vi "Calculate_w12.vi"(0 "Data in":fxp<+/-,32,14>[](array[numeric])=[0.0, 0.0, 0.0, 0.0, 0.0, 0.0, 0.0, 0.0], 1 "w12_a":fxp<+/-,32,12>, 2 "w12_b":fxp<+/-,32,14>, 5 "reset":bool, 11 "valid in":bool, 12 "1/dt":fxp<+/-,32,26>=10000000.0 format="%#_45g", 13 "dw scale":i32, 14 "w12 scale":i32) -> (4 "data out":fxp<+/-,32,14>[](array[numeric]), 6 "dw":fxp<+/-,64,48>, 10 "w12":fxp<+/-,64,48>, 15 "valid out":bool)   [LabVIEW 2025]
uses:
  <vilib>/rvi/FXPMathLib/FxpDiv/subVIs/nifxpmath_Div_SimConfig.ctl
  <vilib>/rvi/FXPMathLib/FxpDiv/simVIs/DllFxpDivTemp_sub.vi
  <vilib>/rvi/FXPMathLib/FxpAdd/XNode/nifxpmath_Add.xnode
  <vilib>/rvi/FXPMathLib/FxpSub/XNode/nifxpmath_Sub.xnode
  <vilib>/rvi/FXPMathLib/FxpMul/XNode/nifxpmath_Multiplier.xnode
  <vilib>/rvi/FXPMathLib/FxpReciprocal/XNode/nifxpmath_Reciprocal.xnode
  <vilib>/rvi/FXPMathLib/FxpDiv/XNode/nifxpmath_Div.xnode
  <vilib>/rvi/FXPMathLib/sim/FxpSim.dll
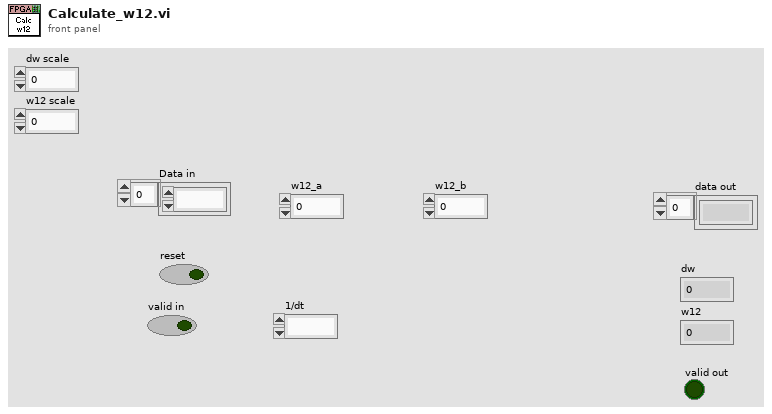
[diagram p1: front panel]
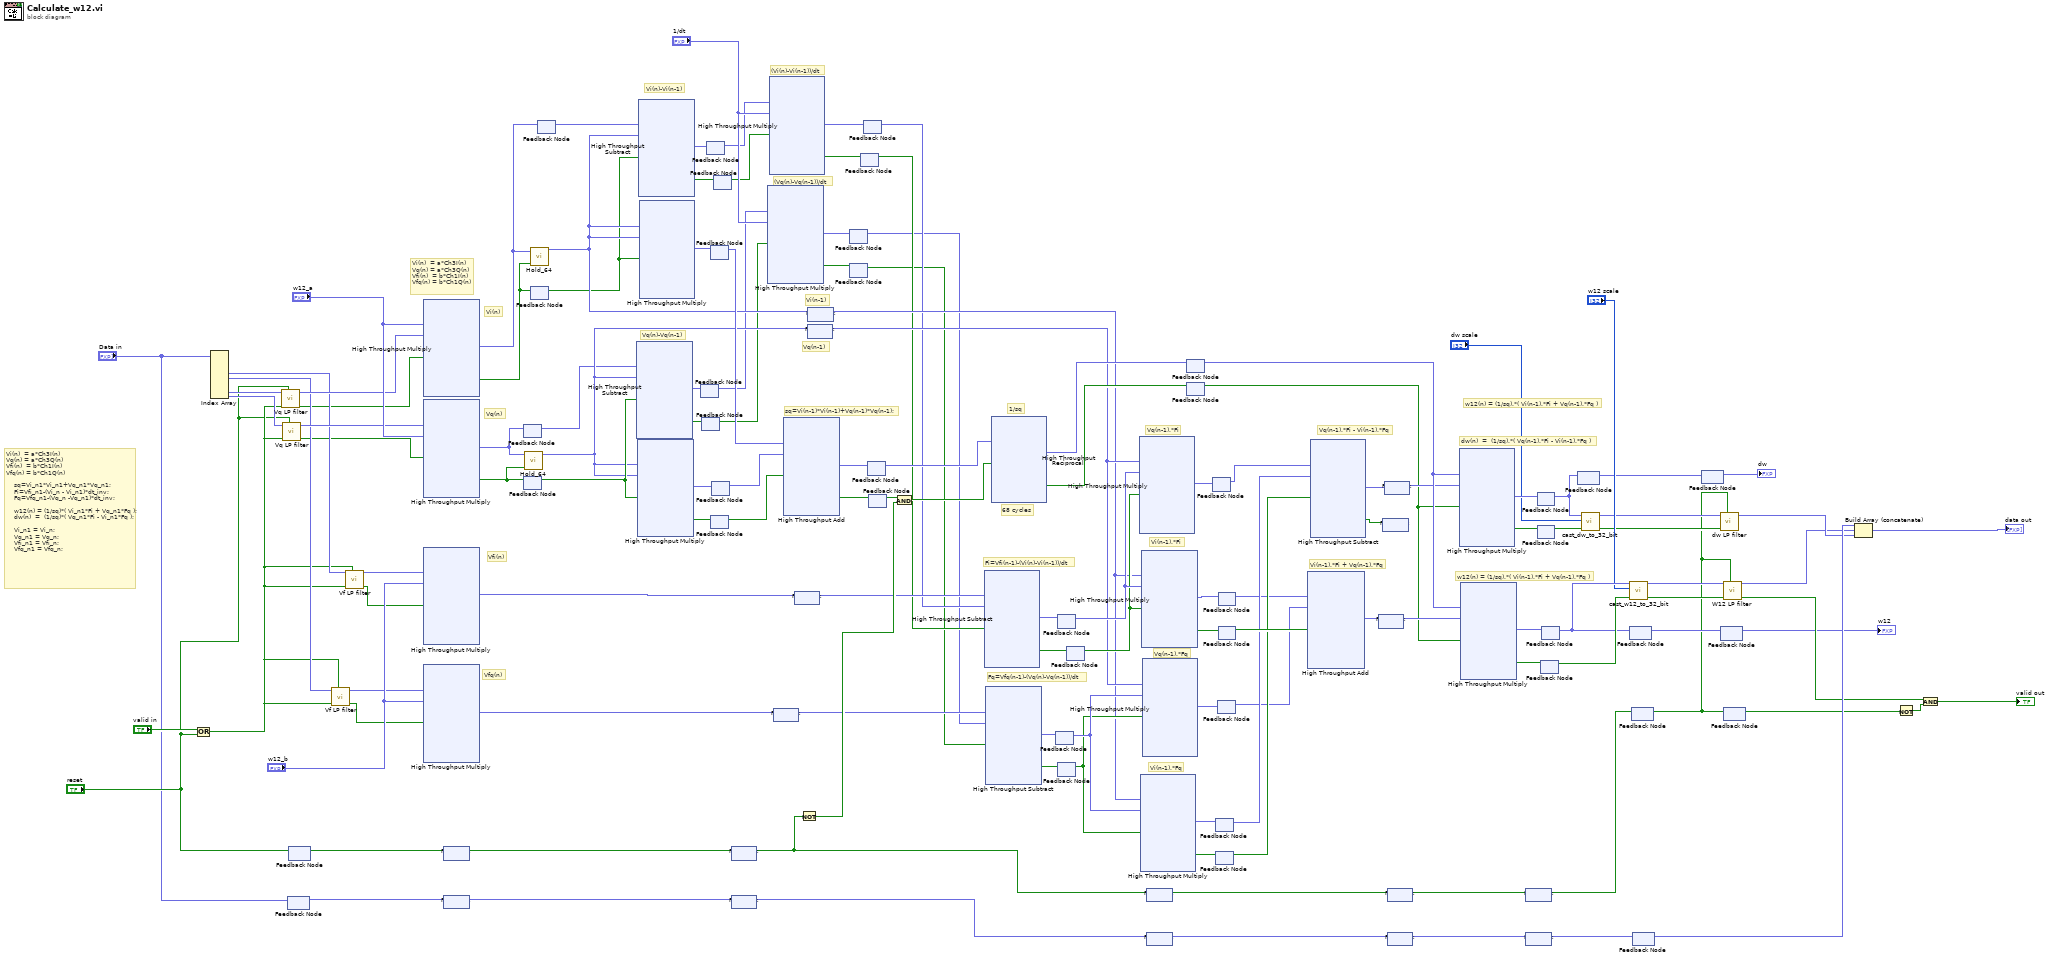
[diagram p0: block diagram]
diagram:
  # "68 cycles"
  # "w12(n) = (1/sq).*( Vi(n-1).*Fi + Vq(n-1).*Fq )"
  # "dw(n)  =  (1/sq).*( Vq(n-1).*Fi - Vi(n-1).*Fq )"
  # "1/sq"
  # "w12(n) = (1/sq).*( Vi(n-1).*Fi + Vq(n-1).*Fq )"
  # "Vq(n-1).*Fi - Vi(n-1).*Fq"
  # "Vi(n-1).*Fi + Vq(n-1).*Fq"
  # "Vi(n-1).*Fq"
  # "Vq(n-1).*Fi"
  # "Vq(n-1).*Fq"
  # "Vq(n-1)"
  # "Vi(n-1)"
  # "Vi(n-1).*Fi"
  # "Fq=Vfq(n-1)-(Vq(n)-Vq(n-1))/dt"
  # "Fi=Vfi(n-1)-(Vi(n)-Vi(n-1))/dt"
  # "(Vq(n)-Vq(n-1))/dt"
  # "(Vi(n)-Vi(n-1))/dt"
  # "Vq(n)-Vq(n-1)"
  # "Vi(n)-Vi(n-1)"
  # "sq=Vi(n-1)*Vi(n-1)+Vq(n-1)*Vq(n-1);"
  # "Vfq(n)"
  # "Vfi(n)"
  # "Vq(n)"
  # "Vi(n)  = a*Ch3I(n)\nVq(n) = a*Ch3Q(n)\nVfi(n)  = b*Ch1I(n)\nVfq(n) = b*Ch1Q(n)"
  # "Vi(n)"
  # "Vi(n)  = a*Ch3I(n)\nVq(n) = a*Ch3Q(n)\nVfi(n)  = b*Ch1I(n)\nVfq(n) = b*Ch1Q(n)\n    \n    sq=Vi_n1*Vi_n1+Vq_n1*Vq_n1;\n    Fi=Vfi_n1-(Vi_n - Vi_n1)*dt_inv;\n    Fq=Vfq_n1-(Vq_n -Vq_n1)*dt_inv;\n    \n    w12(n) = (1/sq)*( Vi_n1*Fi + Vq_n1*Fq );\n    dw(n)  =  (1/sq)*( Vq_n1*Fi - Vi_n1*Fq );\n    \n    Vi_n1 = Vi_n;\n    Vq_n1 = Vq_n;\n    Vfi_n1 = Vfi_n;\n    Vfq_n1 = Vfq_n;"
  n1 = Or(x="valid in", y="reset") -> (x .or. y?=w5:bool)
  n2 = Index Array(array="Data in") -> (element #3=w11:fxp<+/-,32,14>, element #4=w13:fxp<+/-,32,14>, element #7=w17:fxp<+/-,32,14>, element #8=w15:fxp<+/-,32,14>)  [unwired: 8 in, 4 out]
  n3 = call "Vq LP filter.vi"("reset"="reset", "input valid"=w5, "x"=w17) -> ("output valid"=w6:bool, "y"=w16:fxp<+/-,32,14>)  [unwired: 7 in]
  n4 = call "Vq LP filter.vi"("reset"="reset", "input valid"=w5, "x"=w15) -> ("output valid"=w7:bool, "y"=w14:fxp<+/-,32,14>)  [unwired: 7 in]
  n5 = feedback #1() -> (w1:fxp<+/-,32,14>[])  [unwired: 1 in]
  n6 = feedback-in #1("Data in") -> ()
  n7 = feedback #2() -> (w3:bool)  [unwired: 1 in]
  n8 = feedback-in #2("reset") -> ()
  n9 = call "Vf LP filter.vi"("reset"=w5, "input valid"=w5, "x"=w13) -> ("output valid"=w9:bool, "y"=w12:fxp<+/-,32,14>)  [unwired: 7 in]
  n10 = call "Vf LP filter.vi"("reset"=w5, "input valid"=w5, "x"=w11) -> ("output valid"=w8:bool, "y"=w10:fxp<+/-,32,14>)  [unwired: 7 in]
  n11 = xnode ("High Throughput Multiply")("x"="w12_a", "y"=w16, "input valid"=w6) -> ("x*y"=w89:fxp<+/-,64,26>, "output valid"=w88:bool)  [unwired: 1 in, 1 out]
  n12 = xnode ("High Throughput Multiply")("x"=w10, "y"="w12_b", "input valid"=w8) -> ("x*y"=w91:fxp<+/-,64,28>)  [unwired: 1 in, 2 out]
  n13 = xnode ("High Throughput Multiply")("x"=w14, "y"="w12_a", "input valid"=w7) -> ("x*y"=w87:fxp<+/-,64,26>, "output valid"=w86:bool)  [unwired: 1 in, 1 out]
  n14 = xnode ("High Throughput Multiply")("x"=w12, "y"="w12_b", "input valid"=w9) -> ("x*y"=w90:fxp<+/-,64,28>)  [unwired: 1 in, 2 out]
  n15 = feedback #3() -> (w101:bool)  [unwired: 1 in]
  n16 = feedback-in #3(w3) -> ()
  n17 = feedback #4() -> (w100:fxp<+/-,32,14>[])  [unwired: 1 in]
  n18 = feedback-in #4(w1) -> ()
  n19 = feedback #5() -> (w63:fxp<+/-,64,26>)  [unwired: 1 in]
  n20 = feedback-in #5(w87) -> ()
  n21 = feedback #6() -> (w65:bool)  [unwired: 1 in]
  n22 = feedback-in #6(w86) -> ()
  n23 = call "Hold_64.vi"("valid in"=w86, "value in"=w87) -> ("value out"=w64:fxp<+/-,64,26>)  [unwired: 8 in, 1 out]
  n24 = call "Hold_64.vi"("valid in"=w88, "value in"=w89) -> ("value out"=w67:fxp<+/-,64,26>)  [unwired: 8 in, 1 out]
  n25 = feedback #7() -> (w66:bool)  [unwired: 1 in]
  n26 = feedback-in #7(w88) -> ()
  n27 = feedback #8() -> (w72:fxp<+/-,64,26>)  [unwired: 1 in]
  n28 = feedback-in #8(w89) -> ()
  n29 = xnode "High Throughput Subtract"("x"=w63, "y"=w64, "input valid"=w65) -> ("x-y"=w124:fxp<+/-,64,27>, "output valid"=w122:bool)  [unwired: 1 in, 1 out]
  n30 = xnode ("High Throughput Multiply")("x"=w64, "y"=w64, "input valid"=w65) -> ("x*y"=w129:fxp<+/-,64,52>, "output valid"=w121:bool)  [unwired: 1 in, 1 out]
  n31 = xnode "High Throughput Subtract"("x"=w72, "y"=w67, "input valid"=w66) -> ("x-y"=w125:fxp<+/-,64,27>, "output valid"=w123:bool)  [unwired: 1 in, 1 out]
  n32 = xnode ("High Throughput Multiply")("x"=w67, "y"=w67, "input valid"=w66) -> ("x*y"=w128:fxp<+/-,64,52>)  [unwired: 1 in, 2 out]
  n33 = feedback #9() -> (w56:fxp<+/-,64,27>)  [unwired: 1 in]
  n34 = feedback-in #9(w124) -> ()
  n35 = feedback #10() -> (w55:bool)  [unwired: 1 in]
  n36 = feedback-in #10(w122) -> ()
  n37 = feedback #11() -> (w54:fxp<+/-,64,27>)  [unwired: 1 in]
  n38 = feedback-in #11(w125) -> ()
  n39 = feedback #12() -> (w127:fxp<+/-,64,52>)  [unwired: 1 in]
  n40 = feedback-in #12(w128) -> ()
  n41 = feedback #13() -> (w120:bool)  [unwired: 1 in]
  n42 = feedback-in #13(w121) -> ()
  n43 = feedback-in #14(w129) -> ()
  n44 = feedback #14() -> (w126:fxp<+/-,64,52>)  [unwired: 1 in]
  n45 = feedback #15() -> (w53:bool)  [unwired: 1 in]
  n46 = feedback-in #15(w123) -> ()
  n47 = feedback #16() -> (w94:bool)  [unwired: 1 in]
  n48 = feedback-in #16(w101) -> ()
  n49 = feedback #17() -> (w97:fxp<+/-,32,14>[])  [unwired: 1 in]
  n50 = feedback-in #17(w100) -> ()
  n51 = xnode ("High Throughput Multiply")("x"=w56, "y"="1/dt", "input valid"=w55) -> ("x*y"=w116:fxp<+/-,64,44>, "output valid"=w117:bool)  [unwired: 1 in, 1 out]
  n52 = xnode ("High Throughput Multiply")("x"=w54, "y"="1/dt", "input valid"=w53) -> ("x*y"=w119:fxp<+/-,64,44>, "output valid"=w118:bool)  [unwired: 1 in, 1 out]
  n53 = feedback #18() -> (w68:fxp<+/-,64,28>)  [unwired: 1 in]
  n54 = feedback-in #18(w90) -> ()
  n55 = xnode "High Throughput Add"("x"=w127, "y"=w126, "input valid"=w120) -> ("x+y"=w108:fxp<+/-,64,53>, "output valid"=w109:bool)  [unwired: 1 in, 1 out]
  n56 = feedback #19() -> (w69:fxp<+/-,64,28>)  [unwired: 1 in]
  n57 = feedback-in #19(w91) -> ()
  n58 = Not(x=w94) -> (.not. x?=w92:bool)
  n59 = feedback #20() -> (w71:fxp<+/-,64,26>)  [unwired: 1 in]
  n60 = feedback-in #20(w64) -> ()
  n61 = feedback #21() -> (w70:fxp<+/-,64,26>)  [unwired: 1 in]
  n62 = feedback-in #21(w67) -> ()
  n63 = feedback #22() -> (w59:fxp<+/-,64,44>)  [unwired: 1 in]
  n64 = feedback-in #22(w116) -> ()
  n65 = feedback #23() -> (w58:bool)  [unwired: 1 in]
  n66 = feedback-in #23(w117) -> ()
  n67 = feedback #24() -> (w60:bool)  [unwired: 1 in]
  n68 = feedback-in #24(w118) -> ()
  n69 = feedback #25() -> (w61:fxp<+/-,64,44>)  [unwired: 1 in]
  n70 = feedback-in #25(w119) -> ()
  n71 = feedback #26() -> (w83:fxp<+/-,64,53>)  [unwired: 1 in]
  n72 = feedback-in #26(w108) -> ()
  n73 = feedback #27() -> (w95:bool)  [unwired: 1 in]
  n74 = feedback-in #27(w109) -> ()
  n75 = And(x=w95, y=w92) -> (x .and. y?=w93:bool)
  n76 = xnode "High Throughput Subtract"("x"=w69, "y"=w61, "input valid"=w60) -> ("x-y"=w52:fxp<+/-,64,45>, "output valid"=w51:bool)  [unwired: 1 in, 1 out]
  n77 = xnode "High Throughput Subtract"("x"=w68, "y"=w59, "input valid"=w58) -> ("x-y"=w50:fxp<+/-,64,45>, "output valid"=w49:bool)  [unwired: 1 in, 1 out]
  n78 = xnode "High Throughput Reciprocal"("x"=w83, "input valid"=w93) -> ("1/x"=w82:fxp<+/-,64,12>, "output valid"=w107:bool)  [unwired: 1 in, 1 out]
  n79 = feedback #28() -> (w113:fxp<+/-,64,45>)  [unwired: 1 in]
  n80 = feedback-in #28(w50) -> ()
  n81 = feedback #29() -> (w112:bool)  [unwired: 1 in]
  n82 = feedback-in #29(w49) -> ()
  n83 = feedback #30() -> (w115:fxp<+/-,64,45>)  [unwired: 1 in]
  n84 = feedback-in #30(w52) -> ()
  n85 = feedback #31() -> (w114:bool)  [unwired: 1 in]
  n86 = feedback-in #31(w51) -> ()
  n87 = xnode ("High Throughput Multiply")("x"=w71, "y"=w115, "input valid"=w114) -> ("x*y"=w48:fxp<+/-,64,71>)  [unwired: 1 in, 2 out]
  n88 = xnode ("High Throughput Multiply")("x"=w70, "y"=w113, "input valid"=w112) -> ("x*y"=w44:fxp<+/-,64,71>, "output valid"=w43:bool)  [unwired: 1 in, 1 out]
  n89 = xnode ("High Throughput Multiply")("x"=w70, "y"=w115, "input valid"=w114) -> ("x*y"=w47:fxp<+/-,64,71>, "output valid"=w46:bool)  [unwired: 1 in, 1 out]
  n90 = xnode ("High Throughput Multiply")("x"=w71, "y"=w113, "input valid"=w112) -> ("x*y"=w45:fxp<+/-,64,71>)  [unwired: 1 in, 2 out]
  n91 = feedback #32() -> (w85:bool)  [unwired: 1 in]
  n92 = feedback-in #32(w94) -> ()
  n93 = feedback #33() -> (w98:fxp<+/-,32,14>[])  [unwired: 1 in]
  n94 = feedback-in #33(w97) -> ()
  n95 = feedback #34() -> (w57:fxp<+/-,64,12>)  [unwired: 1 in]
  n96 = feedback-in #34(w82) -> ()
  n97 = feedback #35() -> (w37:bool)  [unwired: 1 in]
  n98 = feedback-in #35(w107) -> ()
  n99 = feedback #36() -> (w36:fxp<+/-,64,71>)  [unwired: 1 in]
  n100 = feedback-in #36(w48) -> ()
  n101 = feedback #37() -> (w35:fxp<+/-,64,71>)  [unwired: 1 in]
  n102 = feedback-in #37(w44) -> ()
  n103 = feedback #38() -> (w110:bool)  [unwired: 1 in]
  n104 = feedback-in #38(w43) -> ()
  n105 = feedback #39() -> (w33:fxp<+/-,64,71>)  [unwired: 1 in]
  n106 = feedback-in #39(w45) -> ()
  n107 = feedback #40() -> (w34:fxp<+/-,64,71>)  [unwired: 1 in]
  n108 = feedback-in #40(w47) -> ()
  n109 = feedback #41() -> (w111:bool)  [unwired: 1 in]
  n110 = feedback-in #41(w46) -> ()
  n111 = xnode "High Throughput Add"("x"=w34, "y"=w33, "input valid"=w111) -> ("x+y"=w39:fxp<+/-,64,72>)  [unwired: 1 in, 2 out]
  n112 = xnode "High Throughput Subtract"("x"=w36, "y"=w35, "input valid"=w110) -> ("x-y"=w42:fxp<+/-,64,72>, "output valid"=w41:bool)  [unwired: 1 in, 1 out]
  n113 = feedback #42() -> (w38:fxp<+/-,64,72>)  [unwired: 1 in]
  n114 = feedback-in #42(w39) -> ()
  n115 = feedback #43() -> ()  [unwired: 2 in]
  n116 = feedback-in #43(w41) -> ()
  n117 = feedback #44() -> (w40:fxp<+/-,64,72>)  [unwired: 1 in]
  n118 = feedback-in #44(w42) -> ()
  n119 = feedback #45() -> (w84:bool)  [unwired: 1 in]
  n120 = feedback-in #45(w85) -> ()
  n121 = feedback #46() -> (w99:fxp<+/-,32,14>[])  [unwired: 1 in]
  n122 = feedback-in #46(w98) -> ()
  n123 = xnode ("High Throughput Multiply")("x"=w57, "y"=w40, "input valid"=w37) -> ("x*y"=w106:fxp<+/-,64,48>, "output valid"=w79:bool)  [unwired: 1 in, 1 out]
  n124 = xnode ("High Throughput Multiply")("x"=w57, "y"=w38, "input valid"=w37) -> ("x*y"=w105:fxp<+/-,64,48>, "output valid"=w102:bool)  [unwired: 1 in, 1 out]
  n125 = feedback #47() -> (w75:bool)  [unwired: 1 in]
  n126 = feedback-in #47(w84) -> ()
  n127 = feedback #48() -> (w74:fxp<+/-,32,14>[])  [unwired: 1 in]
  n128 = feedback-in #48(w99) -> ()
  n129 = feedback #49() -> (w77:fxp<+/-,64,48>)  [unwired: 1 in]
  n130 = feedback-in #49(w106) -> ()
  n131 = feedback #50() -> (w78:bool)  [unwired: 1 in]
  n132 = feedback-in #50(w79) -> ()
  n133 = feedback #51() -> (w80:bool)  [unwired: 1 in]
  n134 = feedback-in #51(w102) -> ()
  n135 = feedback #52() -> (w76:fxp<+/-,64,48>)  [unwired: 1 in]
  n136 = feedback-in #52(w105) -> ()
  n137 = feedback #53() -> (w19:fxp<+/-,64,48>)  [unwired: 1 in]
  n138 = feedback-in #53(w77) -> ()
  n139 = call "cast_dw_to_32_bit.vi"("input valid"=w78, "Shift"="dw scale", "x"=w77) -> ("output valid"=w28:bool, "y"=w30:fxp<+/-,32,14>)  [unwired: 7 in]
  n140 = feedback #54() -> (w23:fxp<+/-,64,48>)  [unwired: 1 in]
  n141 = feedback-in #54(w76) -> ()
  n142 = call "cast_w12_to_32_bit.vi"("input valid"=w80, "Shift"="w12 scale", "x"=w76) -> ("output valid"=w26:bool, "y"=w27:fxp<+/-,32,14>)  [unwired: 7 in]
  n143 = feedback #55() -> (w21:bool)  [unwired: 1 in]
  n144 = feedback-in #55(w75) -> ()
  n145 = feedback #56() -> (w73:fxp<+/-,32,14>[])  [unwired: 1 in]
  n146 = feedback-in #56(w74) -> ()
  n147 = feedback #57() -> (→"dw":fxp<+/-,64,48>)  [unwired: 1 in]
  n148 = feedback-in #57(w19) -> ()
  n149 = call "dw LP filter.vi"("reset"=w21, "input valid"=w28, "x"=w30) -> ("y"=w29:fxp<+/-,32,14>)  [unwired: 7 in, 1 out]
  n150 = feedback #58() -> (→"w12":fxp<+/-,64,48>)  [unwired: 1 in]
  n151 = feedback-in #58(w23) -> ()
  n152 = call "W12 LP filter.vi"("reset"=w21, "input valid"=w26, "x"=w27) -> ("output valid"=w24:bool, "y"=w25:fxp<+/-,32,14>)  [unwired: 7 in]
  n153 = feedback #59() -> (w20:bool)  [unwired: 1 in]
  n154 = feedback-in #59(w21) -> ()
  n155 = Build Array (concatenate)(w73, w25, w29) -> (→"data out":fxp<+/-,32,14>[])
  n156 = Not(x=w20) -> (.not. x?=w103:bool)
  n157 = And(x=w24, y=w103) -> (x .and. y?=→"valid out":bool)
